vi "train_cont.vi"(7 "LabVIEW Web Service Request":refnum<class "Web Request.lvclass">) -> ()   [LabVIEW 2014]
uses:
  <vilib>/wsapi/Web Request.lvclass
  DataManager/StateStore/Controls/DataFunction.ctl
panel:
  # "Use the Web Service Request input terminal to call the VIs on the Web Services palette. Do not remove it from the connector pane unless you don't need access to the palette."
  # "Each additional control wired to the connector pane will be available as an input in the URL. To include an indicator in terminal-mode output (the default setting), it must also be wired to the connector pane."
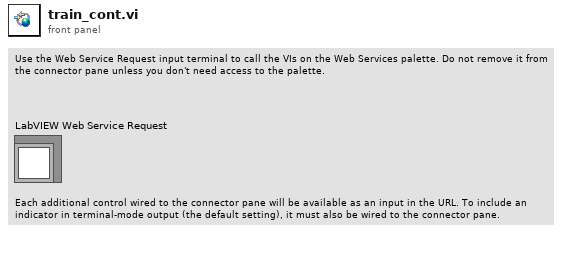
[diagram p1: front panel]
types:
  T1 = typedef "DataFunction.ctl" = enum16{"Initialise", "Release", "Get Data", "Set Data", "Preview Data"}
  T2 = typedef "CData Core Control.ctl" = cluster{"train_data_array":cluster{"uuid":string, "int":i32, "posit_array":cluster{"x":dbl, "y":dbl, "z":dbl}[]}[], "train_control_array":cluster{"uuid":string, "throttle":dbl, "brake":dbl, "horn":dbl, "wait":dbl, "name":string, "mode":string, "dest":string}[], "switch_data_array":cluster{"switch_posit":cluster{"x":dbl, "y":dbl, "z":dbl}, "manual":bool}[], "switch_control_array":cluster{"switch_posit":cluster{"x":dbl, "y":dbl, "z":dbl}, "switch":bool, "invert":bool, "wait":dbl}[]}
  T3 = cluster{"uuid":string, "throttle":dbl, "brake":dbl, "horn":dbl, "wait":dbl, "name":string, "mode":string, "dest":string}[]
  T4 = cluster{"uuid":string, "throttle":dbl, "brake":dbl, "horn":dbl, "wait":dbl, "name":string, "mode":string, "dest":string}
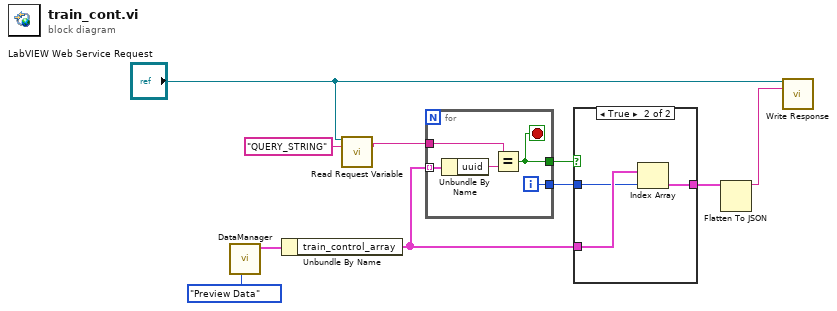
[diagram p0: block diagram]
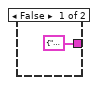
[diagram p2: hidden frame]
diagram:
  n1 = call "DataManager.vi"("DataFunction"=DataFunction."Preview Data") -> ("CData Out"=w9:T2)  [unwired: 9 in, 1 out]
  n2 = Unbundle By Name(w9) -> ("train_control_array"=w6:T3)
  n3 = call <vilib>:"Read Request Variable.vi"("LabVIEW Web Service Request"="LabVIEW Web Service Request", "variable name"="QUERY_STRING") -> ("value"=w4:string)  [unwired: 11 in, 2 out]
  n4 = for {
    tunnel: w6 -> [w15] mode=indexing
    tunnel: w4 -> [w13]
    tunnel: [w12] -> w8
    tunnel: [w11] -> w7
    i -> [w11]
    stop <- w12 stop-if-true
    n5 = Unbundle By Name(w15) -> ("uuid"=w14:string)
    n6 = Equal?(x=w13, y=w14) -> (x = y?=w12:bool)
  }
  n7 = case shown="True" w8 {
    tunnel: w7 -> [_ w18]
    tunnel: w6 -> [_ w19]
    tunnel: [T4 {"uuid"="", "throttle"=0.0, "brake"=0.0, "horn"=0.0, "wait"=0.0, "name"="", "mode"="", "dest"=""} ("train_control") w17] -> w3
    frame False {
    }
    frame True {
      n8 = Index Array(array=w19, index=w18) -> (element=w17:T4)
    }
  }
  n9 = Flatten To JSON(anything=w3) -> (JSON string=w2:string)  [unwired: 2 in, 1 out]
  n10 = call <vilib>:"Write Response.vi"("LabVIEW Web Service Request"="LabVIEW Web Service Request", "response string"=w2) -> ()  [unwired: 12 in, 2 out]
